vi "__goldopt_part1.vi"(8 "f2":dbl, 9 "f1":dbl, 10 "bi":dbl, 11 "ai":dbl) -> (0 "x":dbl, 1 "fout":dbl, 2 "bi 2":dbl, 3 "ai 2":dbl, 4 "f2>f1":bool)   [LabVIEW 2017]
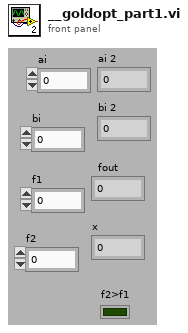
[diagram p1: front panel]
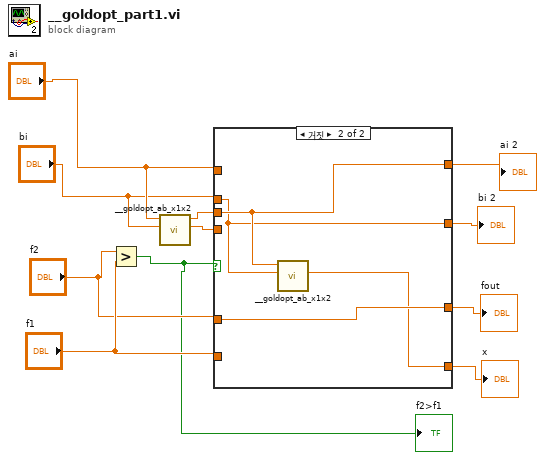
[diagram p0: block diagram]
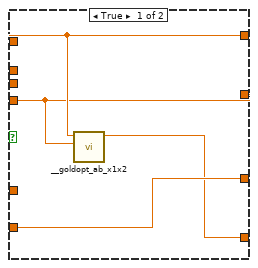
[diagram p2: hidden frame]
diagram:
  n1 = Greater?(x="f2", y="f1") -> (0:w1:bool)
  "f2>f1" <- w1
  n2 = call "__goldopt_ab_x1x2.vi"("bi"="bi", "ai"="ai") -> ("x2"=w8:dbl, "x1"=w4:dbl)  [unwired: 8 in]
  n3 = case shown="거짓" w1 {
    tunnel: "ai" -> [w14 _]
    tunnel: "bi" -> [_ w18]
    tunnel: [w14 w19] -> w2
    tunnel: [w13 w18] -> w9
    tunnel: w8 -> [w13 _]
    tunnel: "f1" -> [w15 _]
    tunnel: [w15 w17] -> w6
    tunnel: [w12 w16] -> w5
    tunnel: w4 -> [_ w19]
    tunnel: "f2" -> [_ w17]
    frame True {
      n4 = call "__goldopt_ab_x1x2.vi"("bi"=w13, "ai"=w14) -> ("x1"=w12:dbl)  [unwired: 8 in, 1 out]
    }
    frame False {
      n5 = call "__goldopt_ab_x1x2.vi"("bi"=w18, "ai"=w19) -> ("x2"=w16:dbl)  [unwired: 8 in, 1 out]
    }
  }
  "bi 2" <- w9
  "fout" <- w6
  "x" <- w5
  "ai 2" <- w2
